vi "OAT Timebase Plot (Unfiltered).vi"(0 "even-angle signals":cluster{"r0":dbl, "dr":dbl, "Y":dbl[]}[](array[cluster]) {"r0" format="%.2p"; "dr" format="%.2p"; "Y" format="%.2f"}, 2 "reset? (F)":bool, 5 "speed profile":T2 {"speed [RPM]" format="%.2f"; "time [s]" format="%.2f"}, 7 "even-angle position info":T3, 9 "revolutions to display [rev]":cluster{"start":dbl, "duration":dbl}={"start"=0.0, "duration"=8.0} {"duration" format="%.2f"; "start" format="%.2f"}, 11 "error in (no error)":errorcluster) -> (4 "x-axis":T1, 6 "y-axis":T1, 15 "error out":errorcluster)   [LabVIEW 2017]
doc: "Draws a timebase plot with unfiltered or filtered data on an XY graph. The unfiltered data comes from the <B>even-angle signals</B> input, the filtered data from the <B>magnitudes</B> and <B>phases [phase lag]</B> inputs. The timebase plot displays the amplitude of a signal as a function of time and marks the tachometer trigger point on the plot. The data type you wire to the <B>even-angle signals</B> input determines the polymorphic instance to use."
uses:
  <vilib>/addons/Sound and Vibration/Order Analysis/Misc/OAT Position Info.ctl
  <vilib>/addons/Sound and Vibration/Order Analysis/Tach Process/SubVIs/speed profile.ctl
  <vilib>/addons/Sound and Vibration/Order Analysis/Backward Compatibility/SubVIs/oa_Timebase Plot Control.ctl
  <vilib>/addons/Sound and Vibration/Order Analysis/Resample Order Tracking/SoundVib_Resampling.lvlib
  <vilib>/addons/Sound and Vibration/Order Analysis/Tach Process/SoundVib_TachProcess.lvlib
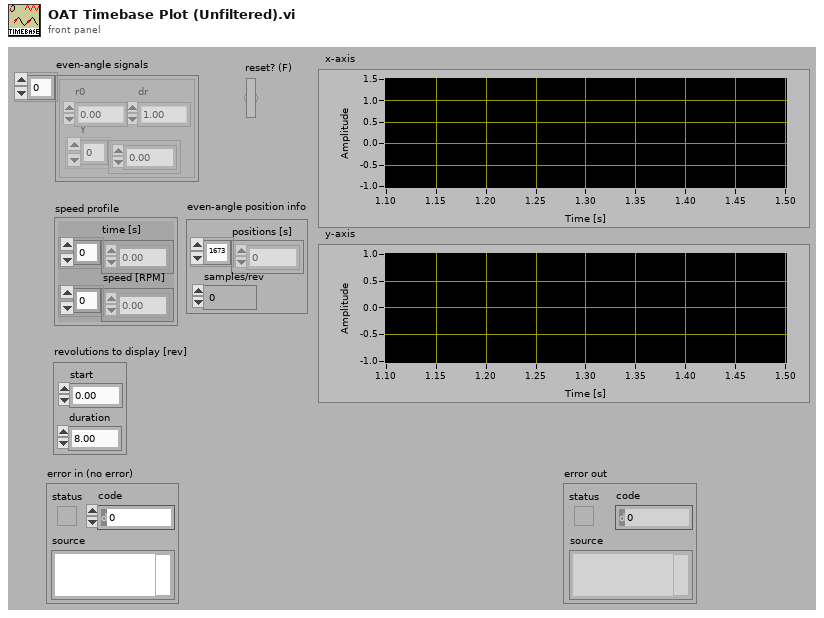
[diagram p1: front panel]
types:
  T1 = typedef "oa_Timebase Plot Control.ctl" = cluster{"X":dbl[], "Y":dbl[]}[]
  T2 = typedef "SoundVib_TachProcess.lvlib/speed profile.ctl" = cluster{"time [s]":dbl[], "speed [RPM]":dbl[]}
  T3 = typedef "OAT Position Info.ctl" = cluster{"positions [s]":dbl[], "samples/rev":dbl}
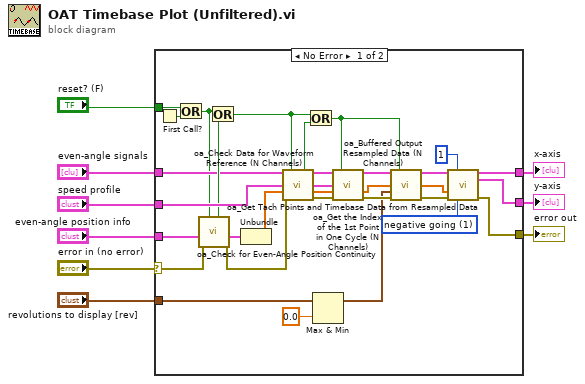
[diagram p0: block diagram]
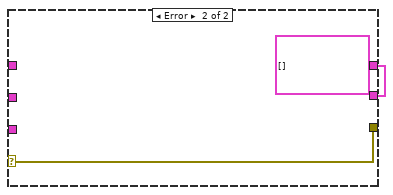
[diagram p2: hidden frame]
diagram:
  n1 = case shown="No Error" "error in (no error)" {
    selector: "error in (no error)" -> [w17 w43]
    tunnel: [w29 w43] -> w8
    tunnel: "even-angle signals" -> [w15 _]
    tunnel: "speed profile" -> [w37 _]
    tunnel: "even-angle position info" -> [w14 _]
    tunnel: "revolutions to display [rev]" -> [w34 _]
    tunnel: [w27 w42] -> w3
    tunnel: [w26 w42] -> w2
    tunnel: "reset? (F)" -> [w10 _]
    frame No Error {
      w20 = u16 1 items=["positive going", "negative going"] ("trigger pulse direction")
      n2 = First Call?() -> (First Call?: T/F=w12:bool)
      n3 = Or(x=w10, y=w12) -> (x .or. y?=w11:bool)
      n4 = call <vilib>:"oa_Check for Even-Angle Position Continuity.vi"("reset in"=w11, "error in (no error)"=w17, "even-angle position info"=w14) -> ("error out"=w16:errorcluster, "even-angle position info dup"=w13:T3, "position not continuous"=w19:bool)  [unwired: 6 in]
      n5 = Or(x=w11, y=w19) -> (x .or. y?=w18:bool)
      n6 = Unbundle(w13) -> ("positions [s]"=w25:dbl[])  [unwired: 1 out]
      n7 = call <vilib>:"oa_Check Data for Waveform Reference (N Channels).vi"("resampled signal"=w15, "reset? (True)"=w18, "speed profile"=w37, "interpolated pulse positions"=w25, "error in (no error)"=w16) -> ("reset"=w36:bool, "resampled data out"=w40:cluster{"r0":dbl, "dr":dbl, "Y":dbl[]}[], "speed profile out"=w38:T2, "interpolated pulse positions out"=w39:dbl[], "error out"=w41:errorcluster)  [unwired: 3 in, 3 out]
      n8 = Or(x=w18, y=w36) -> (x .or. y?=w32:bool)
      n9 = Max & Min(x=w34, y=0.0 ("tach duty")) -> (max(x,y)=w24:cluster{"start":dbl, "duration":dbl})  [unwired: 1 out]
      n10 = call <vilib>:"oa_Get the Index of the 1st Point in One Cycle (N Channels).vi"("resampled signal"=w40, "reset? (True)"=w32, "speed profile"=w38, "interpolated pulse positions"=w39, "error in (no error)"=w41) -> ("resampled signal out"=w35:cluster{"r0":dbl, "dr":dbl, "Y":dbl[]}[], "interpolated pulse positions out"=w22:dbl[], "error out"=w33:errorcluster)  [unwired: 8 in]
      n11 = call <vilib>:"oa_Buffered Output Resampled Data (N Channels).vi"("resampled signal in"=w35, "reset? (True)"=w32, "interpolated pulse positions"=w22, "display revolutions"=w24, "error in"=w33) -> ("resampled signal out"=w31:cluster{"r0":dbl, "dr":dbl, "Y":dbl[]}[], "interpolated pulse positions out"=w21:dbl[], "error out"=w30:errorcluster)  [unwired: 8 in]
      n12 = call <vilib>:"oa_Get Tach Points and Timebase Data from Resampled Data.vi"("resampled signal in"=w31, "tach duty"=1, "interpolated pulse positions [s]"=w21, "error in"=w30, "trigger pulse direction"=w20) -> ("X axis"=w27:cluster{dbl[], dbl[]}[], "Y axis"=w26:cluster{dbl[], dbl[]}[], "error out"=w29:errorcluster)  [unwired: 8 in]
    }
    frame Error {
      w42 = cluster{dbl[], dbl[]}[] [] ("X axis")
    }
  }
  "error out" <- w8
  "y-axis" <- w2
  "x-axis" <- w3
